vi "CSM - Flood of Events Handler Side Loop.vi"() -> ()   [LabVIEW 2020, in "Communicable State Machine.lvlib"]
uses:
  Communicable State Machine.lvlib
panel:
  in  "Slide":dbl(slide) scale=0.0..10.0
  in  "CSM Module":string
  # "Flood of Events:\n\nPanel/Pane Size Event\nSlide/Knob... User Event by dragging\nNumeric Control Value Change Event by Arraw Button"
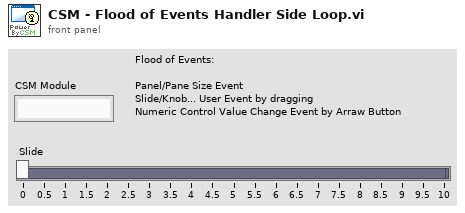
[diagram p1: front panel]
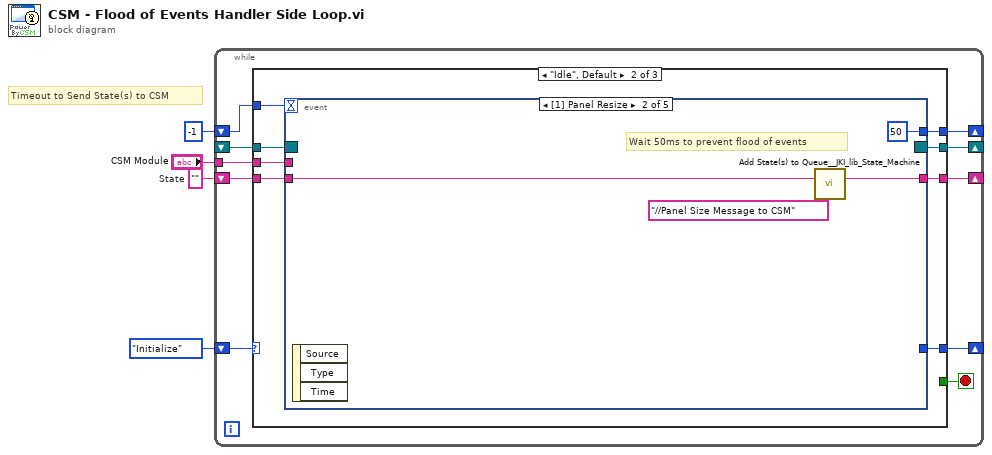
[diagram p0: block diagram]
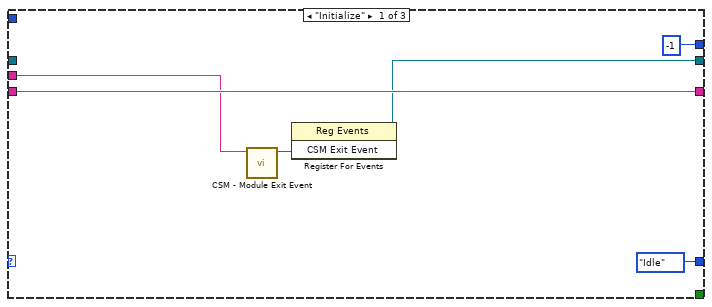
[diagram p2: hidden frame]
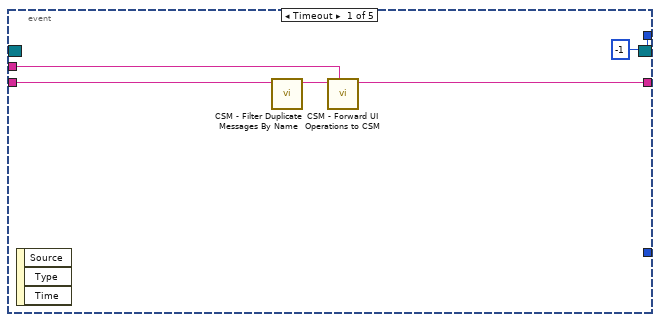
[diagram p3: hidden frame]
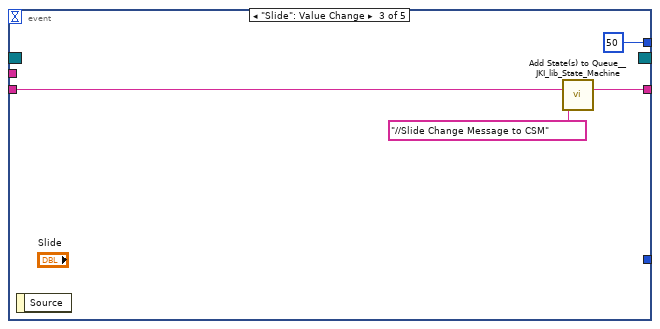
[diagram p4: hidden frame]
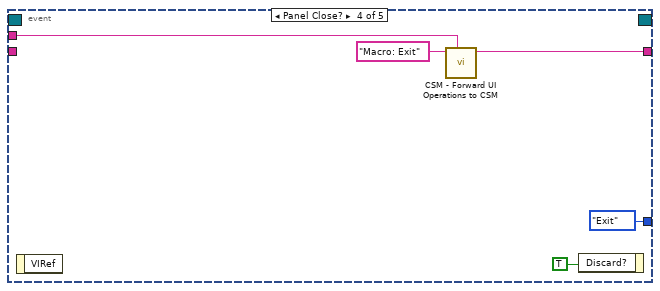
[diagram p5: hidden frame]
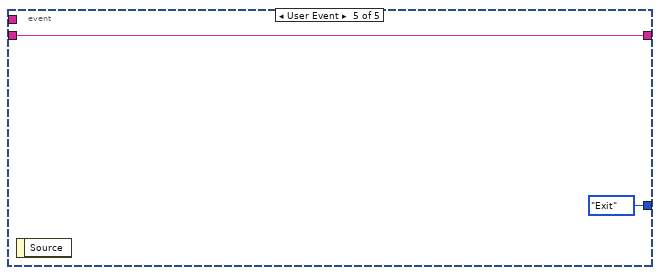
[diagram p6: hidden frame]
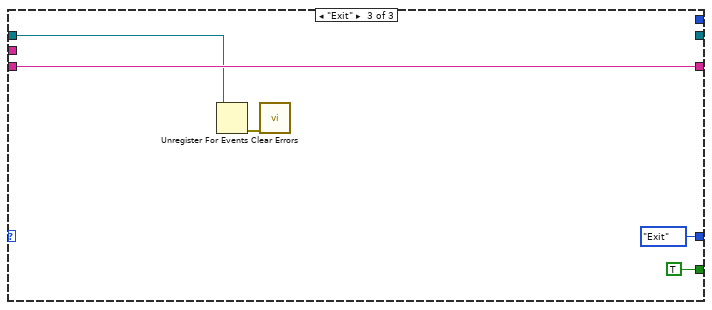
[diagram p7: hidden frame]
diagram:
  w3 = ""  # State
  # "Timeout to Send State(s) to CSM"
  n1 = while {
    shift-right: [w13] -> _
    shift-left: enum16{"Idle", "Initialize", "Exit"}."Initialize" -> [w14]
    tunnel: "CSM Module" -> [w11]
    shift-right: [w9] -> _
    shift-left: w3 -> [w10]
    shift-right: [w7] -> _
    shift-left: -1 -> [w8]
    shift-right: [w6] -> _
    shift-left: _ -> [w5]
    stop <- w12 stop-if-true
    n2 = case shown="\"Idle\", Default" w14 {
      tunnel: [enum16{"Idle", "Initialize", "Exit"}."Idle" w28 enum16{"Idle", "Initialize", "Exit"}."Exit"] -> w13
      tunnel: [_ _ TRUE] -> w12
      tunnel: w11 -> [w16 w27 _]
      tunnel: w10 -> [w19 w25 w51]
      tunnel: [w19 w26 w51] -> w9
      tunnel: w8 -> [_ w23 _]
      tunnel: [-1 w24 _] -> w7
      tunnel: [w15 w21 _] -> w6
      tunnel: w5 -> [_ w22 w50]
      frame "Initialize" {
        n3 = call "CSM - Module Exit Event.vi"("Name(\"\" to use uuid) in"=w16) -> ("CSM Exit Event"=w17:refnum<user-event>)  [unwired: 9 in, 1 out]
        n4 = register-events(w17) -> (reference out=w15:refnum<event-registration>)  [unwired: 2 in, 1 out]
      }
      frame "Idle", Default {
        n5 = event shown="[1] Panel Resize" {
          selector: w22 -> [_ _ _ _ _]
          dyn-events: [_ _ _ _ _] -> w21
          timeout: w23 -> [_ _ _ _ _]
          tunnel: [_ _ _ enum16{"Idle", "Initialize", "Exit"}."Exit" enum16{"Idle", "Initialize", "Exit"}."Exit"] -> w28
          tunnel: w27 -> [w29 _ _ w43 _]
          tunnel: w25 -> [w32 w37 w41 _ w48]
          tunnel: [w30 w36 w40 w42 w48] -> w26
          tunnel: [-1 50 50 _ _] -> w24
          event Timeout {
            n6 = event-data() -> ()  [unwired: 1 in, 3 out]
            n7 = call "CSM - Filter Duplicate Messages By Name.vi"("States"=w32) -> ("States out"=w31:string)  [unwired: 10 in]
            n8 = call "CSM - Forward UI Operations to CSM.vi"("Name(\"\" to use uuid)"=w29, "State(s) in (\"\")"=w31) -> ("States Out"=w30:string)  [unwired: 9 in]
          }
          event Panel Resize {
            # "Wait 50ms to prevent flood of events"
            n9 = event-data() -> ()  [unwired: 1 in, 3 out]
            n10 = call "Add State(s) to Queue__JKI_lib_State_Machine.vi"("State(s) in (\"\")"=w37, "State(s) at Back (\"\")"="//Panel Size Message to CSM" ("State(s) at Back (\"\")")) -> ("States Out"=w36:string)  [unwired: 13 in]
          }
          event "Slide": Value Change {
            n11 = event-data() -> ()  [unwired: 1 in, 1 out]
            n12 = call "Add State(s) to Queue__JKI_lib_State_Machine.vi"("State(s) in (\"\")"=w41, "State(s) at Back (\"\")"="//Slide Change Message to CSM" ("State(s) at Back (\"\")")) -> ("States Out"=w40:string)  [unwired: 13 in]
          }
          event Panel Close? {
            n13 = event-data() -> ()  [unwired: 1 in, 1 out]
            n14 = call "CSM - Forward UI Operations to CSM.vi"("Name(\"\" to use uuid)"=w43, "State(s) in (\"\")"="Macro: Exit" ("State")) -> ("States Out"=w42:string)  [unwired: 9 in]
            n15 = event-data("Discard?"=TRUE) -> ()  [unwired: 1 in, 1 out]
          }
          event User Event {
            n16 = event-data() -> ()  [unwired: 1 in, 1 out]
          }
        }
      }
      frame "Exit" {
        n17 = Unregister For Events(event registration refnum=w50) -> (error out=w49:errorcluster)  [unwired: 1 in]
        n18 = call "Clear Errors.vi"("error in (no error)"=w49) -> ()  [unwired: 5 in, 2 out]
      }
    }
  }
